vi "GEMM_LabVIEW.vi"(7 "Iteration":i32, 11 "Size":i32) -> (3 "Result(s)":dbl format="%.6f")   [LabVIEW 2020]
uses:
  4e24d26d-fcbb-44a5-9aa8-75639d06e416.vi
  <vilib>/Analysis/baseanly.llb/Real A x B.vi
  2ed5783d-9886-4979-abaf-b24675aa47c9.vi
  <vilib>/Utility/High Resolution Relative Seconds.vi
  <vilib>/Analysis/NI_AALBase.lvlib
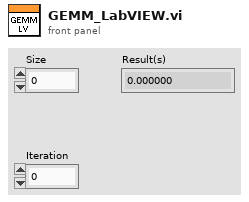
[diagram p1: front panel]
types:
  T1 = typedef "NI_Matrix.lvlib/RealMatrix.ctl" = dbl[][]
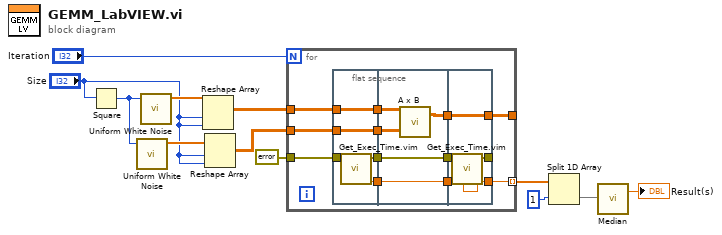
[diagram p0: block diagram]
diagram:
  n1 = Square(x="Size") -> (x^2=w6:i32)
  n2 = call <vilib>:"Uniform White Noise.vi"("samples"=w6) -> ("uniform white noise"=w9:dbl[])  [unwired: 9 in, 1 out]
  n3 = call <vilib>:"Uniform White Noise.vi"("samples"=w6) -> ("uniform white noise"=w10:dbl[])  [unwired: 9 in, 1 out]
  n4 = Reshape Array(w10, "Size", "Size") -> (w8:dbl[][])
  n5 = Reshape Array(w9, "Size", "Size") -> (w12:dbl[][])
  n6 = for {
    N: "Iteration" -> [_]
    tunnel: w8 -> [w24]
    tunnel: errorcluster {"status"=FALSE, "code"=0, "source"=""} ("error out") -> [w22]
    tunnel: [w23] -> _
    tunnel: [w15] -> w11 mode=indexing
    tunnel: w12 -> [w14]
    n7 = flat-sequence {
      tunnel: w22 -> [w28]
      tunnel: w24 -> [w29]
      tunnel: [w29] -> w21
      tunnel: [w27] -> w20
      tunnel: [w26] -> w16
      tunnel: w14 -> [w25]
      tunnel: [w25] -> w13
      tunnel: w21 -> [w34]
      tunnel: w20 -> [w32]
      tunnel: [w33] -> w19
      tunnel: [w32] -> w18
      tunnel: [w31] -> w17
      tunnel: w16 -> [w31]
      tunnel: w13 -> [w30]
      tunnel: [w37] -> _
      tunnel: [w39] -> w23
      tunnel: w19 -> [w39]
      tunnel: w18 -> [w38]
      tunnel: w17 -> [w36]
      tunnel: [w35] -> w15
      frame #0 {
        n8 = call "Get_Exec_Time.vim"("error in (no error)"=w28) -> ("T(n)"=w26:dbl, "error out"=w27:errorcluster)  [unwired: 6 in, 1 out]
      }
      frame #1 {
        n9 = call-poly <vilib>:"A x B.vi"("B"=w30, "A"=w34) -> ("A x B"=w33:T1)  [unwired: 1 out]
      }
      frame #2 {
        n10 = call "Get_Exec_Time.vim"("T(n-1)"=w36, "error in (no error)"=w38) -> ("error out"=w37:errorcluster, "dT"=w35:dbl)  [unwired: 5 in, 1 out]
      }
    }
  }
  n11 = Split 1D Array(array=w11, index=1) -> (second subarray=w1:dbl[])  [unwired: 1 out]
  n12 = call <vilib>:"Median.vi"("X"=w1) -> ("median"=→"Result(s)":dbl)  [unwired: 1 out]
